vi "Exit Manager.vi"(8 "error in (no error)":errorcluster, 9 "uI Refs":T1, 10 "Analysis Queue":refnum<queue>, 11 "Consumer Queue":refnum<queue>) -> (0 "error out":errorcluster)   [LabVIEW 2024]
uses:
  Controls/RVHR - UI Refs.ctl
  Buttons/ML Analysis.ctl
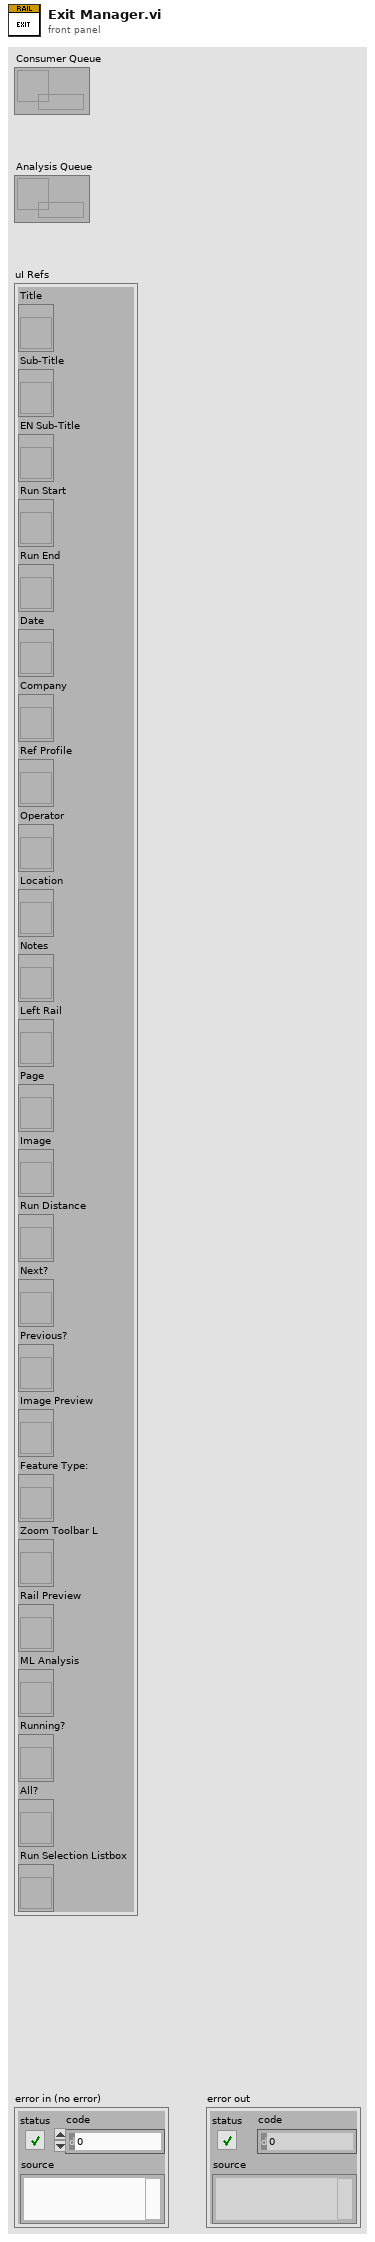
[diagram p1: front panel]
types:
  T1 = typedef "RVHR - UI Refs.ctl" = cluster{"Title":refnum<vi>, "Sub-Title":refnum<vi>, "EN Sub-Title":refnum<vi>, "Run Start":refnum<vi>, "Run End":refnum<vi>, "Date":refnum<vi>, "Company":refnum<vi>, "Ref Profile":refnum<vi>, "Operator":refnum<vi>, "Location":refnum<vi>, "Notes":refnum<vi>, "Left Rail":refnum<vi>, "Page":refnum<vi>, "Image":refnum<vi>, "Run Distance":refnum<vi>, "Next?":refnum<vi>, "Previous?":refnum<vi>, "Image Preview":refnum<vi>, "Feature Type:":refnum<vi>, "Zoom Toolbar L":refnum<vi>, "Rail Preview":refnum<vi>, "ML Analysis":refnum<vi>, "Running?":refnum<vi>, "All?":refnum<vi>, "Run Selection Listbox":refnum<vi>}
  T2 = typedef "ML Analysis.ctl" = bool
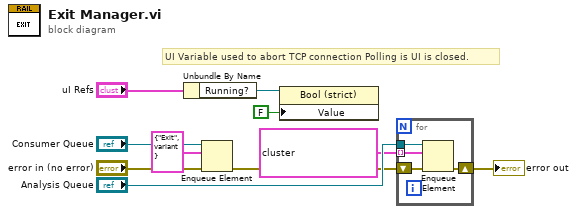
[diagram p0: block diagram]
diagram:
  # "UI Variable used to abort TCP connection Polling is UI is closed."
  n1 = Unbundle By Name("uI Refs") -> ("Running?"=w8:refnum<vi>)
  n2 = Enqueue Element(queue="Consumer Queue", element=cluster{"Command":string, "Data":variant} {"Command"="Exit", "Data"=variant} ("output cluster"), error in (no error)="error in (no error)") -> (error out=w5:errorcluster)  [unwired: 1 in, 2 out]
  n3 = property class="Bool (strict)"(reference=w8, "Value"=T2 FALSE) -> ()  [unwired: 1 in, 2 out]
  n4 = for {
    tunnel: "Analysis Queue" -> [w13]
    tunnel: cluster{"Command":string, "Data":variant}[] [{"Command"="Stop Server", "Data"=variant}, {"Command"="Exit", "Data"=variant}] -> [w11] mode=indexing
    shift-right: [w12] -> w6
    shift-left: w5 -> [w14]
    n5 = Enqueue Element(queue=w13, element=w11, error in (no error)=w14) -> (error out=w12:errorcluster)  [unwired: 1 in, 2 out]
  }
  "error out" <- w6
